vi "Check for Errors.vi"(8 "error in (no error)":errorcluster, 10 "Preceding Items":refnum<class "Item.lvclass">[](array[class]), 11 "Caraya Item in":refnum<class "Caraya Item.lvclass">) -> (0 "error out":errorcluster, 2 "Error User Text":string)   [LabVIEW 2019, in "Caraya Library.lvlib" / "Caraya Item.lvclass"]
doc: "Checks the item for errors. This method is called a lot by the UI, so it should execute quickly.\n\nCopyright: MGI 2016\nAuthor: Derek Trepanier"
uses:
  Caraya Item.lvclass
  libs/Solution.lvlibp/Solution/Item/Item.lvclass
  Caraya Item.lvclass/Caraya Item.ctl
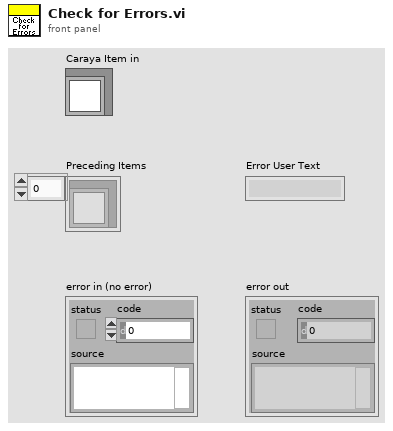
[diagram p1: front panel]
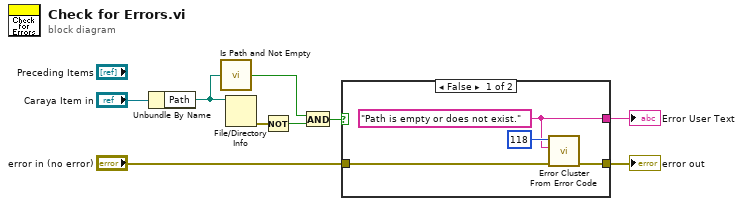
[diagram p0: block diagram]
diagram:
  n1 = Unbundle By Name("Caraya Item in") -> ("Path"=w8:path)
  n2 = call <vilib>:"Is Path and Not Empty.vi"("path"=w8) -> ("Is Path and Not Empty?"=w6:bool)  [unwired: 4 in]
  n3 = File/Directory Info(path=w8) -> (error out=w7:errorcluster)  [unwired: 1 in, 6 out]
  n4 = Not(x=w7) -> (.not. x?=w5:bool)
  n5 = And(x=w6, y=w5) -> (x .and. y?=w1:bool)
  n6 = case shown="False" w1 {
    tunnel: "error in (no error)" -> [w13 w14]
    tunnel: [w12 w14] -> w3
    tunnel: [w10 _] -> w2
    frame False {
      w10 = "Path is empty or does not exist." ("source")
      n7 = call <vilib>:"Error Cluster From Error Code.vi"("error in (no error)"=w13, "error message (\"\")"=w10, "error code (0)"=118) -> ("error out"=w12:errorcluster)  [unwired: 6 in]
    }
    frame True {
    }
  }
  "error out" <- w3
  "Error User Text" <- w2
